vi "NI VeriStand - Add Sections Recursively by Relative Path.vi"(7 "GUID (Default Section)":string="03D3BB89-1485-13A6-56005DE6430FF8B7", 8 "error in":errorcluster, 10 "Relative Section Path":string, 11 "Section Ref in":T1 format="%.0x") -> (0 "error out":errorcluster, 2 "Item Ref":T1 format="%.0x", 3 "Section Ref out":T1 format="%.0x", 4 "Added":bool)   [LabVIEW 2020, in "Custom Device Utility Library.lvlib"]
doc: "Recursively adds sections to a custom device section relative to the item specified by <B>Section Ref in</B>. This VI also sets the GUIDs for the configuration pages to associate with the new sections. If a section with the name you specify already exists, this VI does not overwrite the section."
uses:
  <vilib>/NI VeriStand/Custom Device Tools/Custom Device Utility Library/Custom Device Utility Library.lvlib
  <vilib>/NI VeriStand/Custom Device API/Custom Device Item Ref.ctl
  <vilib>/NI VeriStand/Custom Device Tools/Custom Device Utility Library/NI VeriStand - Ref Constants.vi
  <vilib>/NI VeriStand/Custom Device API/Custom Device API.lvlib
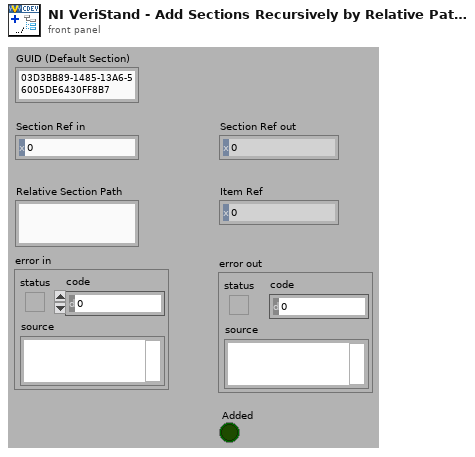
[diagram p1: front panel]
types:
  T1 = typedef "Custom Device API.lvlib/Custom Device Item Ref.ctl" = u64
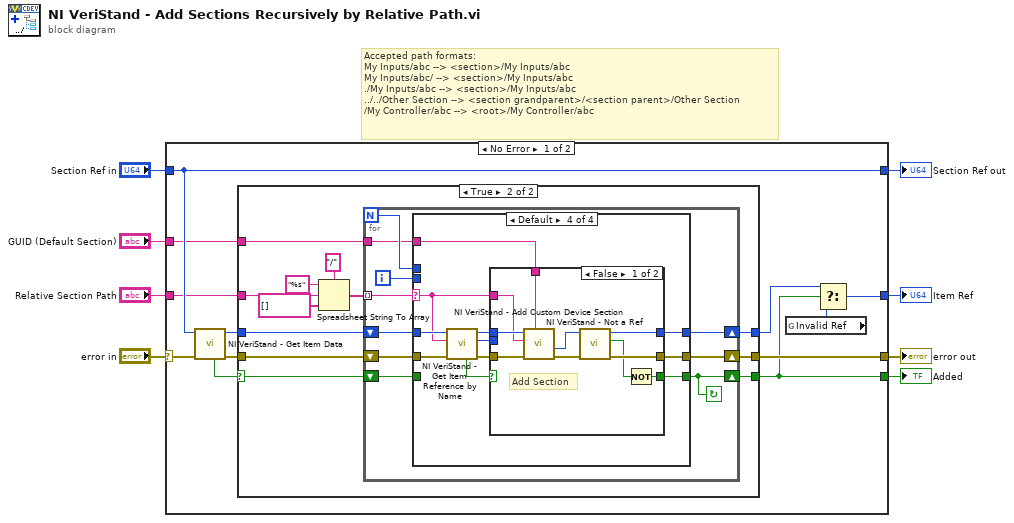
[diagram p0: block diagram]
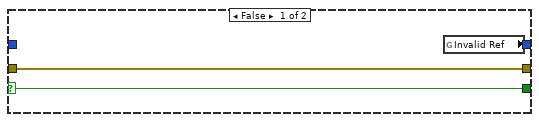
[diagram p2: hidden frame]
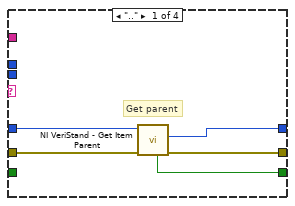
[diagram p3: hidden frame]
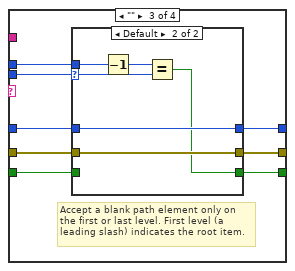
[diagram p5: hidden frame]
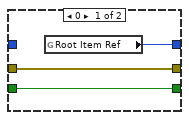
[diagram p6: hidden frame]
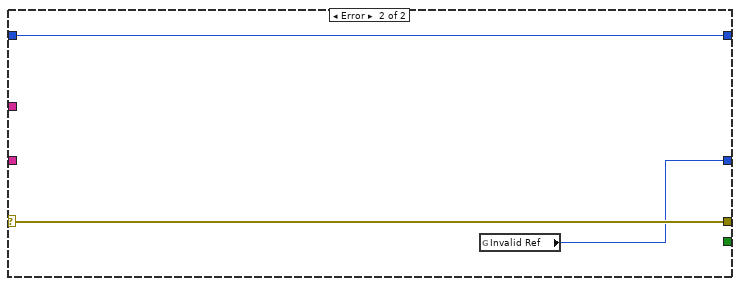
[diagram p8: hidden frame]
diagram:
  # "Accepted path formats:\nMy Inputs/abc --> <section>/My Inputs/abc\nMy Inputs/abc/ --> <section>/My Inputs/abc\n./My Inputs/abc --> <section>/My Inputs/abc\n../../Other Section --> <section grandparent>/<section parent>/Other Section\n/My Controller/abc --> <root>/My Controller/abc"
  n1 = case shown="No Error" "error in" {
    selector: "error in" -> [w14 w97]
    tunnel: [w12 _] -> w8
    tunnel: "Relative Section Path" -> [w18 _]
    tunnel: [w17 w97] -> w6
    tunnel: [w10 w95] -> w5
    tunnel: "Section Ref in" -> [w19 w96]
    tunnel: [w19 w96] -> w2
    tunnel: "GUID (Default Section)" -> [w9 _]
    frame No Error {
      n2 = call <vilib>:"NI VeriStand - Get Item Data.vi"("error in (no error)"=w14, "Item Ref in"=w19) -> ("error out"=w16:errorcluster, "Item Ref out"=w15:T1, "Found"=w13:bool)  [unwired: 7 out]
      n3 = case shown="True" w13 {
        selector: w13 -> [w23 w25]
        tunnel: [w23 w35] -> w12
        tunnel: w18 -> [_ w30]
        tunnel: [w22 w29] -> w17
        tunnel: [w21 w28] -> w11
        tunnel: w16 -> [w22 w27]
        tunnel: w15 -> [_ w26]
        tunnel: w9 -> [_ w24]
        frame False {
          n4 = global read "NI VeriStand - Ref Constants.vi" "Invalid Ref"() -> (w21:T1)
        }
        frame True {
          n5 = Spreadsheet String To Array(delimiter (Tab)="/", format string="%s", spreadsheet string=w30, array type (2D Dbl)=string[] []) -> (array=w34:string[])
          n6 = for {
            N -> [w38]
            shift-right: [w43] -> w28
            shift-left: w26 -> [w44]
            tunnel: w34 -> [w40] mode=indexing
            shift-right: [w42] -> w29
            shift-left: w27 -> [w45]
            shift-right: [w41] -> w35
            shift-left: w25 -> [w37]
            tunnel: w24 -> [w36]
            i -> [w39]
            stop <- w41 continue-if-true
            n7 = case shown="Default" w40 {
              tunnel: w45 -> [w50 w53 w61 w78]
              tunnel: w44 -> [w49 w52 w55 w74]
              tunnel: [w48 w52 w58 w79] -> w43
              tunnel: [w47 w53 w60 w81] -> w42
              tunnel: [w46 w51 w56 w80] -> w41
              tunnel: w39 -> [_ _ w59 _]
              tunnel: w38 -> [_ _ w54 _]
              tunnel: w37 -> [_ w51 w57 _]
              selector: w40 -> [_ _ _ w71]
              tunnel: w36 -> [_ _ _ w72]
              frame ".." {
                # "Get parent"
                n8 = call <vilib>:"NI VeriStand - Get Item Parent.vi"("error in (no error)"=w50, "Item Ref in"=w49) -> ("error out"=w47:errorcluster, "Parent Ref"=w48:T1, "Found"=w46:bool)  [unwired: 7 out]
              }
              frame "." {
                # "Stay at the current level."
              }
              frame "" {
                # "Accept a blank path element only on the first or last level. First level (a leading slash) indicates the root item."
                n9 = case shown="Default" w59 {
                  selector: w59 -> [_ w66]
                  tunnel: w61 -> [w63 w70]
                  tunnel: [w63 w70] -> w60
                  tunnel: [w64 w68] -> w58
                  tunnel: w57 -> [w62 _]
                  tunnel: [w62 w65] -> w56
                  tunnel: w55 -> [_ w68]
                  tunnel: w54 -> [_ w67]
                  frame 0 {
                    n10 = global read "NI VeriStand - Ref Constants.vi" "Root Item Ref"() -> (w64:T1)
                  }
                  frame Default {
                    n11 = Decrement(x=w67) -> (x-1=w69:i32)
                    n12 = Equal?(x=w69, y=w66) -> (x = y?=w65:bool)
                  }
                }
              }
              frame Default {
                n13 = call <vilib>:"NI VeriStand - Get Item Reference by Name.vi"("error in (no error)"=w78, "Item Name"=w71, "Parent Ref in"=w74) -> ("error out"=w76:errorcluster, "Item Ref"=w75:T1, "Parent Ref out"=w73:T1, "Found"=w77:bool)  [unwired: 5 out]
                n14 = case shown="False" w77 {
                  selector: w77 -> [_ w93]
                  tunnel: [w91 w92] -> w81
                  tunnel: [w87 w93] -> w80
                  tunnel: [w86 w94] -> w79
                  tunnel: w72 -> [w85 _]
                  tunnel: w76 -> [w84 w92]
                  tunnel: w75 -> [_ w94]
                  tunnel: w73 -> [w83 _]
                  tunnel: w71 -> [w82 _]
                  frame False {
                    # "Add Section"
                    n15 = call <vilib>:"NI VeriStand - Add Custom Device Section.vi"("GUID (Default Section)"=w85, "error in (no error)"=w84, "Section Name"=w82, "Parent Ref in"=w83) -> ("error out"=w89:errorcluster, "Section Ptr"=w90:T1)  [unwired: 3 in, 3 out]
                    n16 = call <vilib>:"NI VeriStand - Not a Ref.vi"("error in (no error)"=w89, "Item Ref"=w90) -> ("error out"=w91:errorcluster, "Not a Ref"=w88:bool, "Item Ref out"=w86:T1)  [unwired: 7 out]
                    n17 = Not(x=w88) -> (.not. x?=w87:bool)
                  }
                  frame True {
                    # "Item already exists. Don't modify."
                  }
                }
              }
            }
          }
        }
      }
      n18 = global read "NI VeriStand - Ref Constants.vi" "Invalid Ref"() -> (w20:T1)
      n19 = Select(t=w11, s=w12, f=w20) -> (s? t:f=w10:T1)
    }
    frame Error {
      n20 = global read "NI VeriStand - Ref Constants.vi" "Invalid Ref"() -> (w95:T1)
    }
  }
  "Added" <- w8
  "error out" <- w6
  "Section Ref out" <- w2
  "Item Ref" <- w5
